vi "Read Stream.vi"(6 "Timout (s)":i32, 8 "error in (no error)":errorcluster, 9 "Output ref":refnum<vi>, 10 "reader":refnum<k24>, 11 "stream":refnum<k24>) -> (0 "error out":errorcluster)   [LabVIEW 2016, in "LabSSH.lvlib"]
uses:
  LabSSH.lvlib
  C:/Users/thosman/Documents/Development/Labview/ssh in labview/LabSSH/LabSSH/References/Renci.SshNet.dll
  LabSSH/LabSSH/References/Renci.SshNet.dll
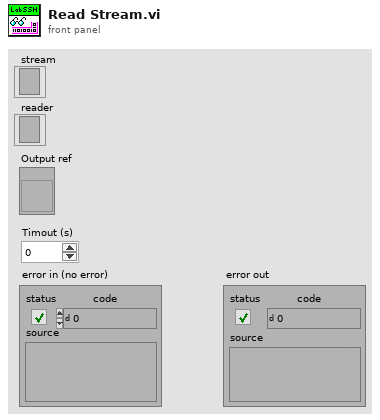
[diagram p1: front panel]
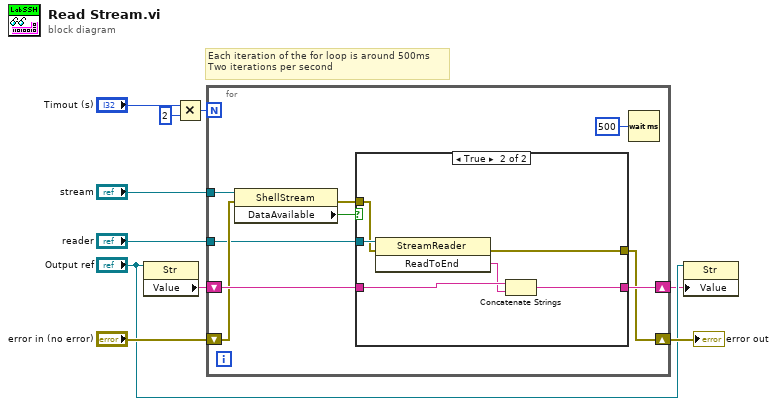
[diagram p0: block diagram]
diagram:
  # "Each iteration of the for loop is around 500ms\nTwo iterations per second"
  n1 = property class="Str"(reference="Output ref") -> ("Value"=w3:string)  [unwired: 1 in, 2 out]
  n2 = Multiply(x="Timout (s)", y=2) -> (x*y=w9:i32)
  n3 = for {
    N: w9 -> [_]
    tunnel: "stream" -> [w18]
    tunnel: "reader" -> [w14]
    shift-right: [w12] -> w1
    shift-left: w3 -> [w16]
    shift-right: [w11] -> w4
    shift-left: "error in (no error)" -> [w15]
    n4 = property class="ShellStream"(reference=w18, error in=w15) -> (error out=w13:errorcluster, "DataAvailable"=w17:bool)  [unwired: 1 out]
    n5 = case shown="True" w17 {
      tunnel: w16 -> [w21 w25]
      tunnel: w14 -> [_ w27]
      tunnel: w13 -> [w20 w26]
      tunnel: [w21 w23] -> w12
      tunnel: [w20 w22] -> w11
      frame False {
      }
      frame True {
        n6 = invoke class="StreamReader" method="ReadToEnd"(reference=w27, error in=w26) -> (error out=w22:errorcluster, "ReadToEnd"=w24:string)  [unwired: 1 in, 1 out]
        n7 = Concatenate Strings(w25, w24) -> (w23:string)
      }
    }
    n8 = Wait (ms)(milliseconds to wait=u32 500) -> ()  [unwired: 1 out]
  }
  "error out" <- w4
  n9 = property class="Str"(reference="Output ref", "Value"=w1) -> ()  [unwired: 1 in, 2 out]
